vi "set laser timing.vi"(7 "timebase":u16, 8 "error in (no error)":errorcluster, 9 "pulse2":u16, 10 "pulse1":u16, 11 "halfperiod":u16) -> (0 "error out":errorcluster)   [LabVIEW 2015, in "SCANalone4x64.lvlib"]
doc: "__declspec(dllimport) void __stdcall set_laser_timing(unsigned short halfperiod, unsigned short pulse1, unsigned short pulse2, unsigned short timebase);"
uses:
  <userlib>/SCANalone4x64/SCANalone4x64.lvlib
  <userlib>/SCANalone4x64/SCANalone4x64.dll
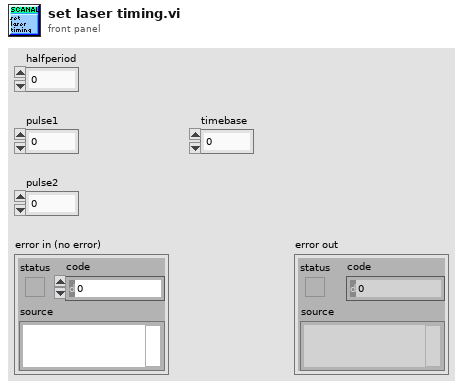
[diagram p1: front panel]
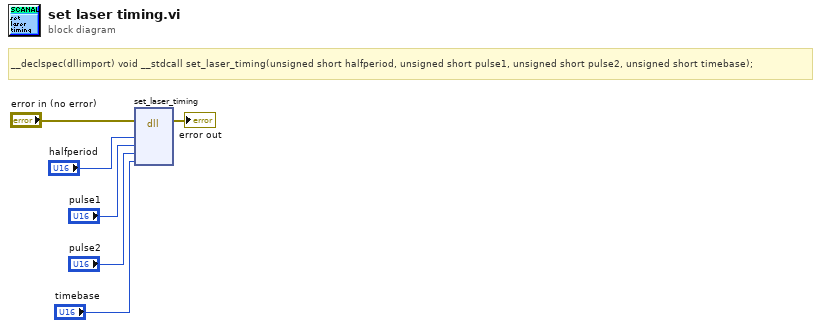
[diagram p0: block diagram]
diagram:
  # "__declspec(dllimport) void __stdcall set_laser_timing(unsigned short halfperiod, unsigned short pulse1, unsigned short pulse2, unsigned short timebase);"
  n1 = dll-call lib="C:/Program Files/National Instruments/LabVIEW 2015/user.lib/SCANalone4x64/SCANalone4x64.*" fn="set_laser_timing"(error in="error in (no error)", "halfperiod"="halfperiod", "pulse1"="pulse1", "pulse2"="pulse2", "timebase"="timebase") -> (error out=→"error out":errorcluster)  [unwired: 7 in, 1 out]
